vi "ssa.vi"(8 "per":dbl, 10 "array 2":dbl[](array[numeric]), 11 "array":dbl[](array[numeric])) -> (3 "motors speed":dbl[](array[numeric]))   [LabVIEW 2015]
uses:
  <vilib>/imath/engines/lvmath2/RunTimeEngine/NodeEndStatement/NIMS_NodeEndStatement_Output.vi
  <instcachedir>/0/NIMS_NodeEndStatement_Output_53EC0D466D134D7ABD903AC30B43404B.lvgen/NIMS_NodeEndStatement_Output_53EC0D466D134D7ABD903AC30B43404B_001.vi
  <vilib>/imath/engines/lvmath2/RunTimeEngine/ErrorHandling/NIMS_Finalize Error.vi
panel:
  out "element":dbl
  out "x+y":dbl[](array[numeric])
  in  "V":dbl=12.0
  in  "Kv":dbl=2100.0
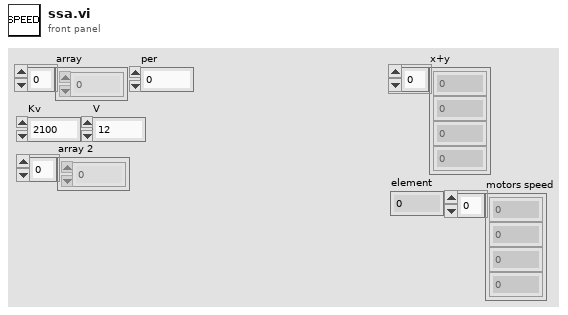
[diagram p1: front panel]
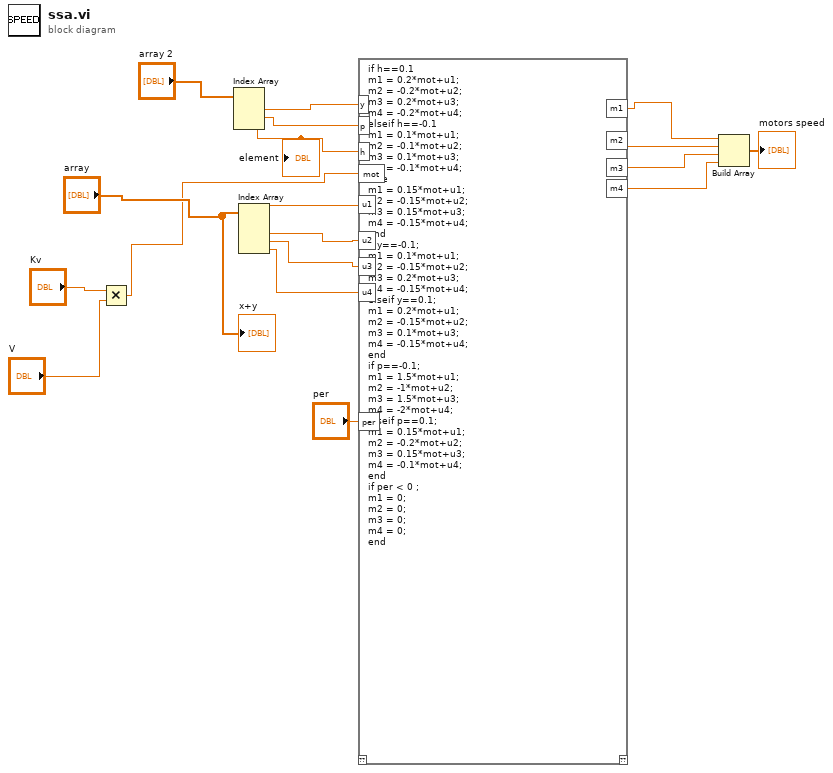
[diagram p0: block diagram]
diagram:
  n1 = Multiply(x="Kv", y="V") -> (x*y=w7:dbl)
  n2 = Index Array ("Index Array 5")(array="array 2") -> (element #1=w11:dbl, element #2=w10:dbl, element #3=w9:dbl)  [unwired: 3 in]
  "element" <- w9
  n3 = Index Array ("Index Array 5")(array="array") -> (element #1=w18:dbl, element #2=w17:dbl, element #3=w16:dbl, element #4=w15:dbl)  [unwired: 4 in]
  n4 = mathscript code="if h==0.1\nm1 = 0.2*mot+u1;\nm2 = -0.2*mot+u2;\nm3 = 0.2*mot+u3;\nm4 = -0.2*mot+u4;\nelseif h==-0.1\nm1 = 0.1*mot+u1;\nm2 = -0.1*mot+u2;\nm3 = 0.1*mot+u3;\nm4 = -0.1*mot+u4;\nelse\nm1 = 0.15*mot+u1;\nm2 = -0.15*mot+u2;\nm3 = 0.15*mot+u3;\nm4 = -0.15*mot+u4;\nend\nif y==-0.1;\nm1 = 0.1*mot+u1;\nm2 = -0.15*mot+u2;\nm3 = 0.2*mot+u3;\nm4 = -0.15*mot+u4;\nelseif y==0.1;\nm1 = 0.2*mot+u1;\nm2 = -0.15*mot+u2;\nm3 = 0.1*mot+u3;\nm4 = -0.15*mot+u4;\nend\nif p==-0.1;\nm1 = 1.5*mot+u1;\nm2 = -1*mot+u2;\nm3 = 1.5*mot+u3;\nm4 = -2*mot+u4;\nelseif p==0.1;\nm1 = 0.15*mot+u1;\nm2 = -0.2*mot+u2;\nm3 = 0.15*mot+u3;\nm4 = -0.1*mot+u4;\nend\nif per < 0 ;\nm1 = 0;\nm2 = 0;\nm3 = 0;\nm4 = 0;\nend"("u1"=w18, "u2"=w17, "u3"=w16, "u4"=w15, "y"=w11, "p"=w10, "h"=w9, "mot"=w7, "per"="per") -> ("m1"=w6:dbl, "m2"=w5:dbl, "m3"=w4:dbl, "m4"=w3:dbl)  [unwired: 1 in, 1 out]
  n5 = Build Array(w6, w5, w4, w3) -> (→"motors speed":dbl[])
  "x+y" <- "array"
